vi "Frame_Drop_Analyzer.vi"() -> ()   [LabVIEW 2020]
uses:
  e96a6f05-e239-40d6-8c1b-574c530f2788.vi
panel:
  out "Lost Frame Num":i32
  out "Duplicated Frame Num":i32
  out "Last Frame Index":u64
  out "First Frame Index":u64
  out "Frame Num":i32
  out "Frame Count":u64[](array[numeric])
  in  "Camera Type":enum16{"4K", "2K"}(ring)
  in  "emb tdms Path":path
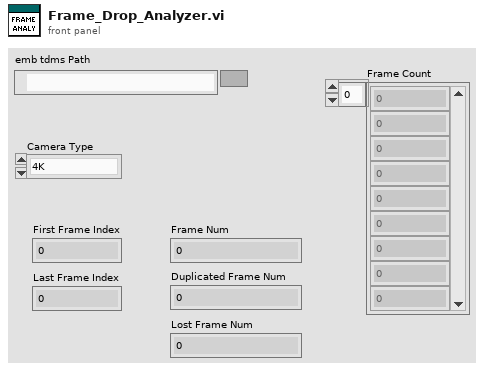
[diagram p1: front panel]
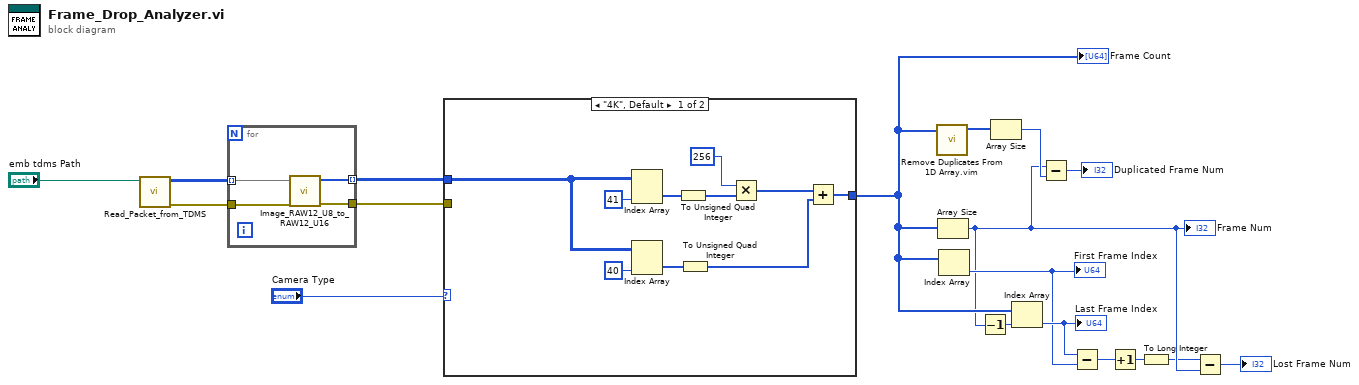
[diagram p0: block diagram]
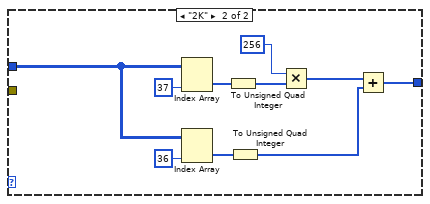
[diagram p2: hidden frame]
diagram:
  n1 = call "Read_Packet_from_TDMS.vi"("TDMS File path"="emb tdms Path") -> ("error out"=w16:errorcluster, "Line Packet Payload"=w17:u8[][])  [unwired: 8 in, 1 out]
  n2 = for {
    tunnel: w17 -> [w22] mode=indexing
    tunnel: w16 -> [w21]
    tunnel: [w20] -> w14 mode=indexing
    tunnel: [w19] -> w13
    n3 = call "Image_RAW12_U8_to_RAW12_U16.vi"("error in (no error)"=w21, "RAW12 Frame (U8)"=w22) -> ("error out"=w19:errorcluster, "RAW12 Frame (U16)"=w20:u16[])  [unwired: 8 in]
  }
  n4 = case shown="\"4K\", Default" "Camera Type" {
    tunnel: w14 -> [w23 w41]
    tunnel: w13 -> [_ _]
    tunnel: [w24 w33] -> w11
    frame "4K", Default {
      n5 = Index Array(array=w23, index (col)=41 ("disabled index (col)")) -> (element=w30:u16[])  [unwired: 1 in]
      n6 = Index Array(array=w23, index (col)=40 ("disabled index (col)")) -> (element=w27:u16[])  [unwired: 1 in]
      n7 = To Unsigned Quad Integer(1:w30) -> (0:w28:u64[])
      n8 = To Unsigned Quad Integer(1:w27) -> (0:w25:u64[])
      n9 = Multiply(x=u64 256, y=w28) -> (x*y=w26:u64[])
      n10 = Add(x=w26, y=w25) -> (x+y=w24:u64[])
    }
    frame "2K" {
      n11 = Index Array(array=w41, index (col)=37 ("disabled index (col)")) -> (element=w39:u16[])  [unwired: 1 in]
      n12 = Index Array(array=w41, index (col)=36 ("disabled index (col)")) -> (element=w36:u16[])  [unwired: 1 in]
      n13 = To Unsigned Quad Integer(1:w39) -> (0:w37:u64[])
      n14 = To Unsigned Quad Integer(1:w36) -> (0:w34:u64[])
      n15 = Multiply(x=u64 256, y=w37) -> (x*y=w35:u64[])
      n16 = Add(x=w35, y=w34) -> (x+y=w33:u64[])
    }
  }
  "Frame Count" <- w11
  n17 = call "Remove Duplicates From 1D Array.vim"("array"=w11) -> ("array with duplicates removed"=w10:u64[])  [unwired: 10 in]
  n18 = Array Size(array=w11) -> (size(s)=w3:i32)
  "Frame Num" <- w3
  n19 = Index Array(array=w11) -> (element=w6:u64)  [unwired: 1 in]
  "First Frame Index" <- w6
  n20 = Decrement(x=w3) -> (x-1=w12:i32)
  n21 = Array Size(array=w10) -> (size(s)=w9:i32)
  n22 = Index Array(array=w11, index=w12) -> (element=w7:u64)
  "Last Frame Index" <- w7
  n23 = Subtract(x=w3, y=w9) -> (x-y=→"Duplicated Frame Num":i32)
  n24 = Subtract(x=w7, y=w6) -> (x-y=w5:u64)
  n25 = Increment(x=w5) -> (x+1=w4:u64)
  n26 = To Long Integer(number=w4) -> (32bit integer=w2:i32)
  n27 = Subtract(x=w2, y=w3) -> (x-y=→"Lost Frame Num":i32)
